vi "DrawVessels.vi"(8 "error in (no error)":errorcluster, 11 "Image in":refnum<class "Image.lvclass">) -> (0 "error out":errorcluster, 3 "Image out":refnum<class "Image.lvclass">)   [LabVIEW 2011, in "Image.lvclass"]
uses:
  Image.lvclass
  Image.lvclass/Image.ctl
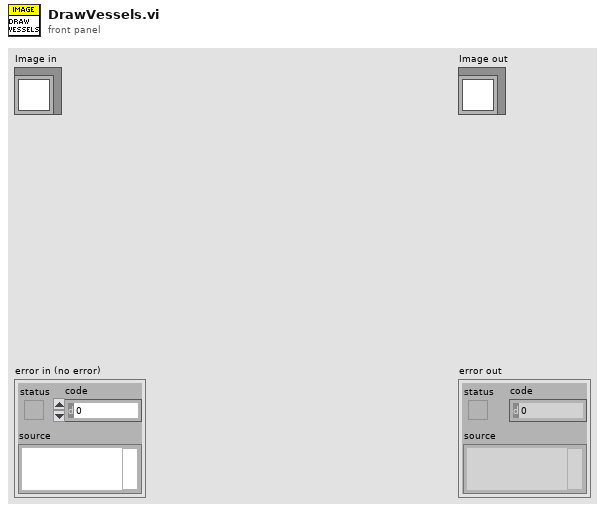
[diagram p1: front panel]
types:
  T1 = typedef "IMAQ Image.ctl" = refnum<image>
  T2 = cluster{"scan_idx":i32, "lens":i32, "mag":dbl, "x":dbl, "y":dbl, "mouse_id":i32, "exp_date":string, "file_name":string, "file_path":path}
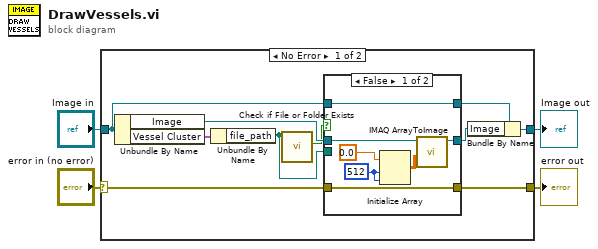
[diagram p0: block diagram]
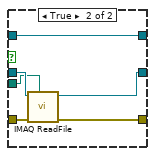
[diagram p2: hidden frame]
diagram:
  n1 = case shown="No Error" "error in (no error)" {
    selector: "error in (no error)" -> [w13 w29]
    tunnel: [w12 w29] -> w3
    tunnel: [w6 w28] -> w1
    tunnel: "Image in" -> [w9 w28]
    frame No Error {
      n2 = Unbundle By Name(w9) -> ("Image"=w14:T1, "Vessel Cluster"=w8:T2)
      n3 = Unbundle By Name(w8) -> ("file_path"=w10:path)
      n4 = call <vilib>:"Check if File or Folder Exists.vi"("path"=w10) -> ("file or folder exists?"=w11:bool)  [unwired: 8 in, 2 out]
      n5 = case shown="False" w11 {
        tunnel: w14 -> [w16 w27]
        tunnel: w13 -> [w20 w26]
        tunnel: [w20 w25] -> w12
        tunnel: w10 -> [_ w24]
        tunnel: w9 -> [w21 w23]
        tunnel: [w21 w23] -> w7
        tunnel: [w17 w22] -> w5
        frame False {
          w18 = 512 ("dimension size")
          n6 = Initialize Array(0.0 ("element"), w18, w18) -> (w15:dbl[][])
          n7 = call "IMAQ ArrayToImage"("Image Pixels (I16)"=w15, "Image"=w16) -> ("Image Out"=w17:T1)  [unwired: 8 in, 1 out]
        }
        frame True {
          n8 = call "IMAQ ReadFile"("File Path"=w24, "error in (no error)"=w26, "Image"=w27) -> ("error out"=w25:errorcluster, "Image Out"=w22:T1)  [unwired: 2 in, 5 out]
        }
      }
      n9 = Bundle By Name(cluster=w7, "Image"=w5) -> (w6:refnum<class "Image.lvclass">)
    }
    frame Error {
    }
  }
  "error out" <- w3
  "Image out" <- w1
